vi "Remote Time Check for Continuous Connection.vi"(7 "Tolerance (2 ms)":u32=2, 8 "error in (no error)":errorcluster, 9 "Number of Attempts (5)":u32=5, 11 "connection ID":refnum<k5>) -> (0 "error out":errorcluster, 1 "Windows OS Up Time (ms)":u32, 2 "Remote OS Up Time (ms)":u32, 3 "connection ID (duplicate)":refnum<k5>)   [LabVIEW 2010, in "Core SubVIs.lvlib"]
doc: "Checks the OS Up Time of a remote computer over a TCP connection."
uses:
  Core SubVIs.lvlib
  TYPE - Remote Time Check State Control.ctl
panel:
  out "Number of Attempts":u32
  out "Valid Trip Time":bool
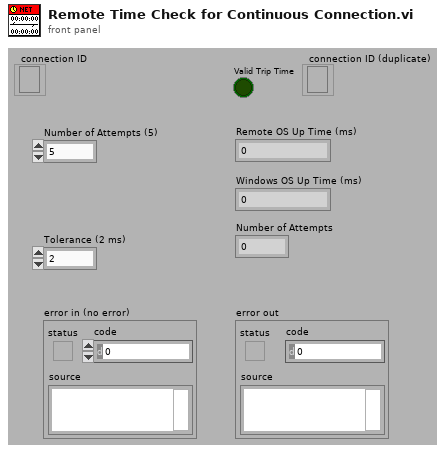
[diagram p1: front panel]
types:
  T1 = typedef "Core SubVIs.lvlib/TYPE - Remote Time Check State Control.ctl" = enum16{"Default", "Open Connection", "Check Time", "Close Connection", "Cleanup"}
  T2 = enum16{"Standard", "Buffered", "CRLF", "Immediate"}
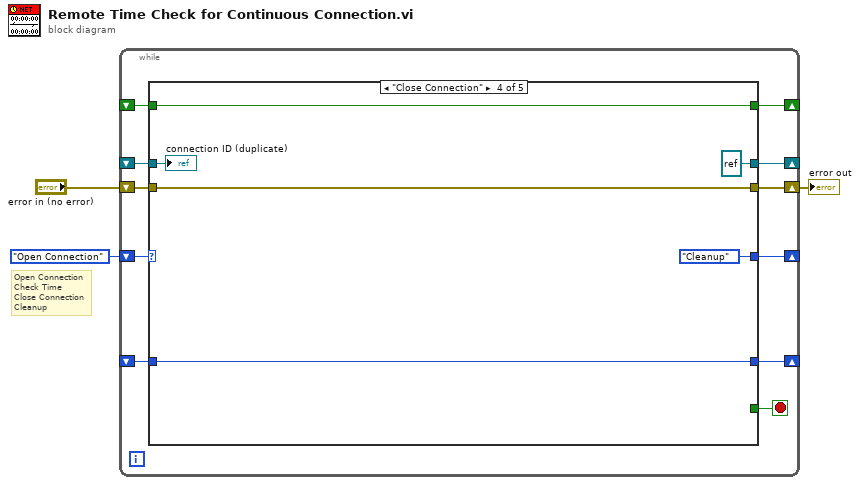
[diagram p0: block diagram]
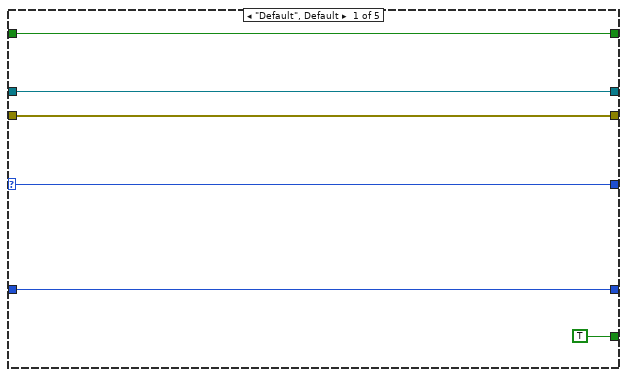
[diagram p2: hidden frame]
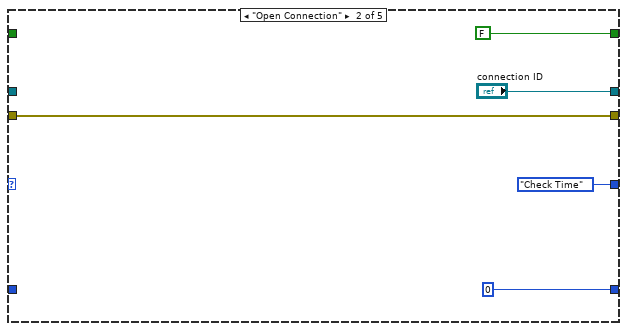
[diagram p3: hidden frame]
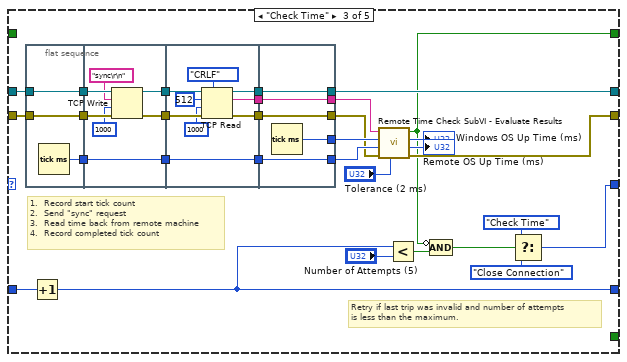
[diagram p4: hidden frame]
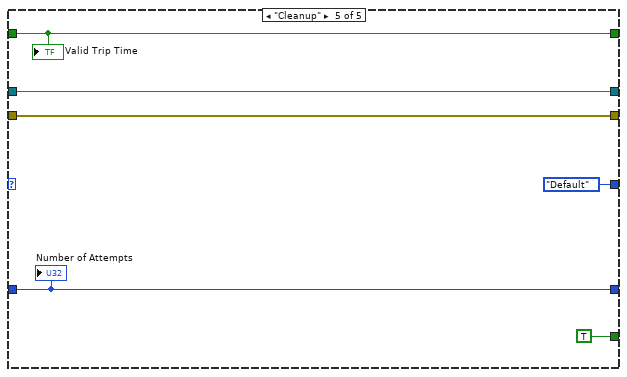
[diagram p5: hidden frame]
diagram:
  # "Open Connection\nCheck Time\nClose Connection\nCleanup"
  n1 = while {
    shift-right: [w13] -> _
    shift-left: TYPE_-_Remote_Time_Check_State_Control."Open Connection" ("State") -> [w14]
    shift-right: [w10] -> w1
    shift-left: "error in (no error)" -> [w9]
    shift-right: [w11] -> _
    shift-left: _ -> [w8]
    shift-right: [w7] -> _
    shift-left: _ -> [w6]
    shift-right: [w5] -> _
    shift-left: _ -> [w4]
    stop <- w12 stop-if-true
    n2 = case shown="\"Close Connection\"" w14 {
      selector: w14 -> [w19 _ _ _ _]
      tunnel: [w19 TYPE_-_Remote_Time_Check_State_Control."Check Time" ("State") w27 TYPE_-_Remote_Time_Check_State_Control."Cleanup" ("State") TYPE_-_Remote_Time_Check_State_Control."Default" ("State")] -> w13
      tunnel: [TRUE _ _ _ TRUE] -> w12
      tunnel: [w16 "connection ID" w43 refnum<k5> refnum ("connection ID") w91] -> w11
      tunnel: [w15 w22 w38 w81 w90] -> w10
      tunnel: w9 -> [w15 w22 w54 w81 w90]
      tunnel: w8 -> [w16 _ w55 w80 w91]
      tunnel: [w18 u32 0 w32 w82 w89] -> w7
      tunnel: w6 -> [w18 _ w34 w82 w89]
      tunnel: [w17 FALSE ("Valid Trip Time") w26 w85 w86] -> w5
      tunnel: w4 -> [w17 _ _ w85 w86]
      frame "Default", Default {
      }
      frame "Open Connection" {
      }
      frame "Check Time" {
        # "Retry if last trip was invalid and number of attempts\nis less than the maximum."
        # "1.  Record start tick count\n2.  Send \"sync\" request\n3.  Read time back from remote machine\n4.  Record completed tick count"
        n3 = flat-sequence {
          tunnel: w55 -> [w58]
          tunnel: w54 -> [w57]
          tunnel: [w58] -> w53
          tunnel: [w57] -> w52
          tunnel: [w56] -> w51
          tunnel: w53 -> [w65]
          tunnel: w52 -> [w62]
          tunnel: w51 -> [w64]
          tunnel: [w63] -> w50
          tunnel: [w64] -> w49
          tunnel: [w61] -> w48
          tunnel: w50 -> [w74]
          tunnel: w49 -> [w73]
          tunnel: w48 -> [w69]
          tunnel: [w72] -> w47
          tunnel: [w73] -> w46
          tunnel: [w67] -> w45
          tunnel: [w66] -> w44
          tunnel: [w76] -> w41
          tunnel: [w77] -> w39
          tunnel: [w78] -> w42
          tunnel: [w79] -> w43
          tunnel: w47 -> [w79]
          tunnel: w46 -> [w78]
          tunnel: w45 -> [w77]
          tunnel: w44 -> [w76]
          tunnel: [w75] -> w40
          frame #0 {
            n4 = Tick Count (ms)() -> (millisecond timer value=w56:u32)
          }
          frame #1 {
            n5 = TCP Write(connection ID=w65, data in="sync\r\n", error in (no error)=w62, 9:1000 ("timeout ms (25000)")) -> (connection ID out=w63:refnum<k5>, error out=w61:errorcluster)  [unwired: 1 out]
          }
          frame #2 {
            n6 = TCP Read(connection ID=w74, bytes to read=512, error in (no error)=w69, 7:T2."CRLF" ("mode (standard)"), 9:1000 ("timeout ms (25000)")) -> (connection ID out=w72:refnum<k5>, data out=w66:string, error out=w67:errorcluster)
          }
          frame #3 {
            n7 = Tick Count (ms)() -> (millisecond timer value=w75:u32)
          }
        }
        n8 = Increment(x=w34) -> (x+1=w32:u32)
        n9 = call "Remote Time Check SubVI - Evaluate Results.vi"("Tolerance (ms)"="Tolerance (2 ms)", "error in (no error)"=w39, "Start Tick Count (ms)"=w42, "Completion Tick Count (ms)"=w40, "Remote Time String (ms)"=w41) -> ("error out"=w38:errorcluster, "Remote OS Up Time (ms)"=→"Remote OS Up Time (ms)":u32, "Windows OS Up Time (ms)"=→"Windows OS Up Time (ms)":u32, "Valid Trip Time"=w26:bool)  [unwired: 3 in]
        n10 = Less?(x=w32, y="Number of Attempts (5)") -> (x < y?=w33:bool)
        n11 = Compound Arithmetic op=AND(invert w26, w33) -> (w30:bool)
        n12 = Select(t=TYPE_-_Remote_Time_Check_State_Control."Check Time" ("State"), s=w30, f=TYPE_-_Remote_Time_Check_State_Control."Close Connection" ("State")) -> (s? t:f=w27:T1)
      }
      frame "Close Connection" {
        "connection ID (duplicate)" <- w80
      }
      frame "Cleanup" {
        "Valid Trip Time" <- w86
        "Number of Attempts" <- w89
      }
    }
  }
  "error out" <- w1
